vi "Level Meter Device (Read).vi"(6 "ISOBUS address":T11=-1 caption="ISOBUS address (-1)", 8 "error in":errorcluster, 11 "Mercury Reference In":T12) -> (0 "error out":errorcluster, 2 "LVL Device Settings":T2, 3 "Mercury Reference Out":T12, 4 "Valid?":T1)   [LabVIEW 2013, in "Mercury iXX.lvlib" / "Level Meter.lvlib"]
doc: "Read the current device configuration for the selected level meter device."
uses:
  <instrlib>/Mercury iXX/Public/Libraries/Level Meter.lvlib
  <instrlib>/Mercury iXX/Public/Controls/Mercury Reference.ctl
  <instrlib>/Mercury iXX/Public/Controls/Comms Transport Layer.ctl
  <instrlib>/Mercury iXX/Private/Controls/Query Dynamic Reference.ctl
  <instrlib>/Mercury iXX/Public/Controls/ISOBus Address.ctl
  <instrlib>/Mercury iXX/Public/Libraries/Level Meter/Controls/Level Meter (Read).ctl
  <instrlib>/Mercury iXX/Public/Controls/Manufacturing Data.ctl
  <instrlib>/Mercury iXX/Public/Libraries/Level Meter/Controls/Nitrogen Configuration.ctl
  <instrlib>/Mercury iXX/Public/Libraries/Level Meter/Controls/Frequency Configuration.ctl
  <instrlib>/Mercury iXX/Public/Libraries/Level Meter/Controls/Signals.ctl
  <instrlib>/Mercury iXX/Public/Libraries/Level Meter/Controls/Helium Configuration.ctl
  <instrlib>/Mercury iXX/Public/Libraries/Level Meter/Controls/Resistance Configuration.ctl
  <instrlib>/Mercury iXX/Public/Libraries/Level Meter/Controls/Pre-Pulse.ctl
  <instrlib>/Mercury iXX/Public/Libraries/Level Meter/Controls/Pulse.ctl
  <instrlib>/Mercury iXX/Public/Controls/Is Valid LED.ctl
  <instrlib>/Mercury iXX/Private/Controls/Command Verbs.ctl
  <instrlib>/Mercury iXX/Mercury iXX.lvlib
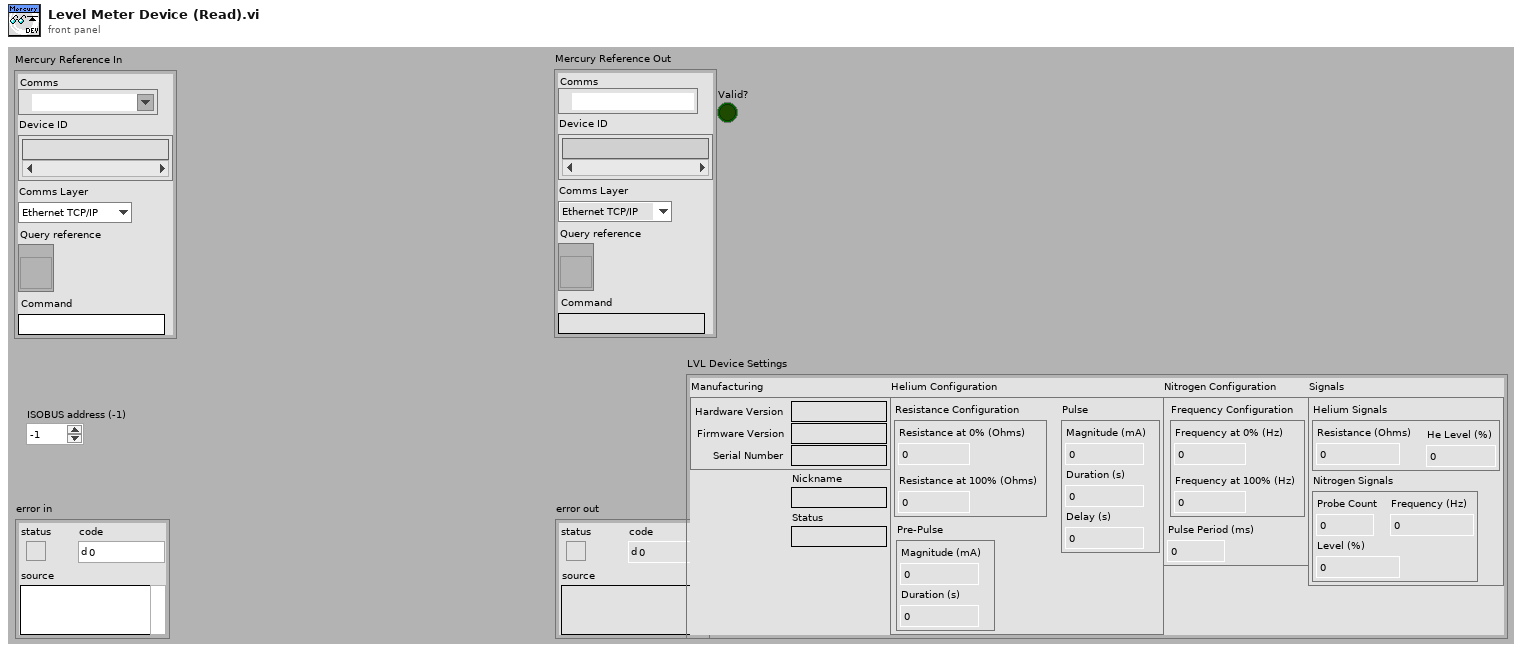
[diagram p1: front panel]
types:
  T1 = typedef "Mercury iXX.lvlib/Is Valid LED.ctl" = bool
  T2 = typedef "Mercury iXX.lvlib/Level Meter.lvlib/Level Meter (Read).ctl" = cluster{"Manufacturing":T3, "Nitrogen Configuration":T4, "Signals":T6, "Nickname":string, "Status":string, "Helium Configuration":T7}
  T3 = typedef "Mercury iXX.lvlib/Manufacturing Data.ctl" = cluster{"Hardware Version":string, "Firmware Version":string, "Serial Number":string}
  T4 = typedef "Mercury iXX.lvlib/Level Meter.lvlib/Nitrogen Configuration.ctl" = cluster{"Frequency Configuration":T5, "Pulse Period":dbl}
  T5 = typedef "Mercury iXX.lvlib/Level Meter.lvlib/Frequency Configuration.ctl" = cluster{"Freq 0%":dbl, "Freq 100%":dbl}
  T6 = typedef "Mercury iXX.lvlib/Level Meter.lvlib/Signals.ctl" = cluster{"Helium Signals":cluster{"Resistance":dbl, "Level":dbl}, "Nitrogen Signals":cluster{"Count":dbl, "Freq":dbl, "Level":dbl}}
  T7 = typedef "Mercury iXX.lvlib/Level Meter.lvlib/Helium Configuration.ctl" = cluster{"Resistance Configuration":T8, "Pre-Pulse":T9, "Pulse":T10}
  T8 = typedef "Mercury iXX.lvlib/Level Meter.lvlib/Resistance Configuration.ctl" = cluster{"Res 0%":dbl, "Res 100%":dbl}
  T9 = typedef "Mercury iXX.lvlib/Level Meter.lvlib/Pre-Pulse.ctl" = cluster{"Magnitude":dbl, "Duration":dbl}
  T10 = typedef "Mercury iXX.lvlib/Level Meter.lvlib/Pulse.ctl" = cluster{"Magnitude":dbl, "Duration":dbl, "Delay":dbl}
  T11 = typedef "Mercury iXX.lvlib/ISOBus Address.ctl" = i32
  T12 = typedef "Mercury iXX.lvlib/Mercury Reference.ctl" = cluster{"Comms":refnum<visa-resource-name>, "Device ID":string[], "Comms Layer":T13, "Command":string, "Query reference":T14}
  T13 = typedef "Mercury iXX.lvlib/Comms Transport Layer.ctl" = enum16{"Ethernet TCP/IP", "USB", "ISOBus - RS-232", "GPIB"}
  T14 = typedef "Mercury iXX.lvlib/Query Dynamic Reference.ctl" = refnum<vi>
  T15 = typedef "Mercury iXX.lvlib/Command Verbs.ctl" = string
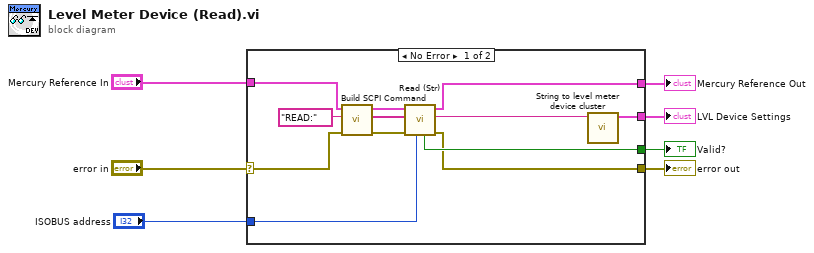
[diagram p0: block diagram]
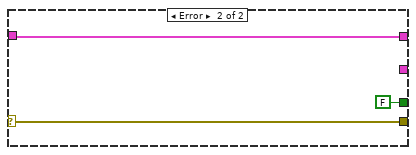
[diagram p2: hidden frame]
diagram:
  n1 = case shown="No Error" "error in" {
    selector: "error in" -> [w10 w21]
    tunnel: "ISOBUS address" -> [w15 _]
    tunnel: [w14 T1 FALSE ("Valid?")] -> w2
    tunnel: "Mercury Reference In" -> [w13 w22]
    tunnel: [w12 w22] -> w4
    tunnel: [w11 w21] -> w1
    tunnel: [w8 _] -> w3
    frame No Error {
      n2 = call <instrlib>:"Build SCPI Command.vi"("error in"=w10, "Verb"=T15 "READ:", "Mercury Reference In"=w13) -> ("error out"=w17:errorcluster, "SCPI Message(s)"=w18:string[], "Mercury Reference Out"=w19:T12)  [unwired: 1 in, 5 out]
      n3 = call <instrlib>:"Read (Str).vi"("ISOBUS address"=w15, "error in"=w17, "SCPI Message(s)"=w18, "Mercury Reference In"=w19) -> ("error out"=w11:errorcluster, "Response"=w9:string, "Mercury Reference Out"=w12:T12, "Valid?"=w14:T1)  [unwired: 4 out]
      n4 = call <instrlib>:"String to level meter device cluster.vi"("LVL Device Details"=w9) -> ("Level Meter"=w8:T2)  [unwired: 10 out]
    }
    frame Error {
    }
  }
  "Mercury Reference Out" <- w4
  "error out" <- w1
  "LVL Device Settings" <- w3
  "Valid?" <- w2
